vi "1ToV.vi"(10 "In1":string) -> (2 "OutV":string)   [LabVIEW 2012]
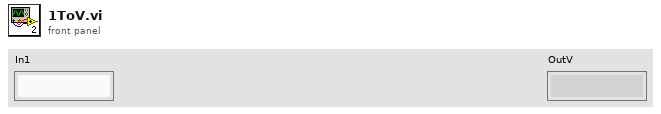
[diagram p1: front panel]
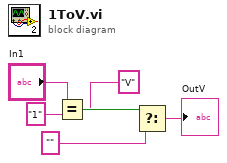
[diagram p0: block diagram]
diagram:
  n1 = Equal?(x="In1", y="1") -> (x = y?=w5:bool)
  n2 = Select(t="V", s=w5, f="") -> (s? t:f=→"OutV":string)
